vi "AVI Video-Limit number of frames.vi"(1 "Frame Size":u32) -> (0 "Limit number of frames":u32)   [LabVIEW 2017]
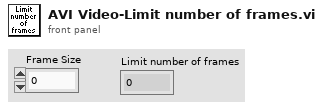
[diagram p1: front panel]
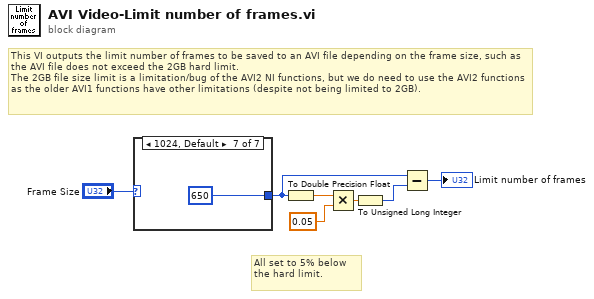
[diagram p0: block diagram]
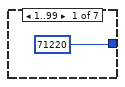
[diagram p2: hidden frame]
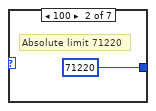
[diagram p3: hidden frame]
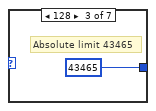
[diagram p4: hidden frame]
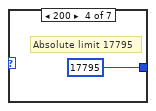
[diagram p5: hidden frame]
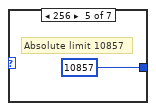
[diagram p6: hidden frame]
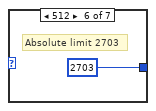
[diagram p7: hidden frame]
diagram:
  # "This VI outputs the limit number of frames to be saved to an AVI file depending on the frame size, such as the AVI file does not exceed the 2GB hard limit.\nThe 2GB file size limit is a limitation/bug of the AVI2 NI functions, but we do need to use the AVI2 functions as the older AVI1 functions have other limitations (despite not being limited to 2GB)."
  # "All set to 5% below the hard limit."
  n1 = case shown="1024, Default" "Frame Size" {
    tunnel: [u32 71220 ("Number of frames") u32 71220 ("Number of frames") u32 43465 ("Number of frames") u32 17795 ("Number of frames") u32 10857 ("Number of frames") u32 2703 ("Number of frames") u32 650 ("Number of frames")] -> w4
    frame 1..99 {
    }
    frame 100 {
      # "Absolute limit 71220"
    }
    frame 128 {
      # "Absolute limit 43465"
    }
    frame 200 {
      # "Absolute limit 17795"
    }
    frame 256 {
      # "Absolute limit 10857"
    }
    frame 512 {
      # "Absolute limit 2703"
    }
    frame 1024, Default {
    }
  }
  n2 = To Double Precision Float(number=w4) -> (double precision float=w7:dbl)
  n3 = Multiply(x=w7, y=0.05) -> (x*y=w6:dbl)
  n4 = To Unsigned Long Integer(number=w6) -> (unsigned 32bit integer=w3:u32)
  n5 = Subtract(x=w4, y=w3) -> (x-y=→"Limit number of frames":u32)
